vi "tack_point_builder.vi"(0 "Boat Location":T1 {"North" format="%#_10f"; "East" format="%#_8f"}, 1 "Loop counts":i32, 2 "Amount to extend tack waypoints (m)":dbl, 5 "Distance for tack to travel (m)":dbl, 7 "Tolerance (meters?)":dbl, 9 "Angle (Final leyline -> WP) (deg)":dbl, 11 "Angle (Other leyline -> WP) (deg)":dbl, 12 "Final leyline (deg)":dbl, 13 "Other leyline (deg)":dbl) -> (4 "Proposed WP array":refnum<class "Waypoint.lvclass">[](array[class]), 6 "Other leyline (deg)":dbl, 10 "Angle (Final leyline -> WP) (deg) OUT":dbl, 15 "Angle (Other leyline -> WP) (deg) OUT":dbl)   [LabVIEW 2013]
doc: "This VI takes the information to build a series of tack waypoints and makes a temporary array of the waypoints.\n\nTHIS VI ASSUMES THAT ANOTHER SHORT TACK WILL BE COMPLETED AFTER IT, IT ENDS ON 'OTHER LEYLINE', NOT FINAL LEYLINE'.s\n\nEric Schneider, September 2014"
uses:
  Data/TypeDefs/UTM Location.ctl
  Classes/Waypoint/Waypoint.lvclass
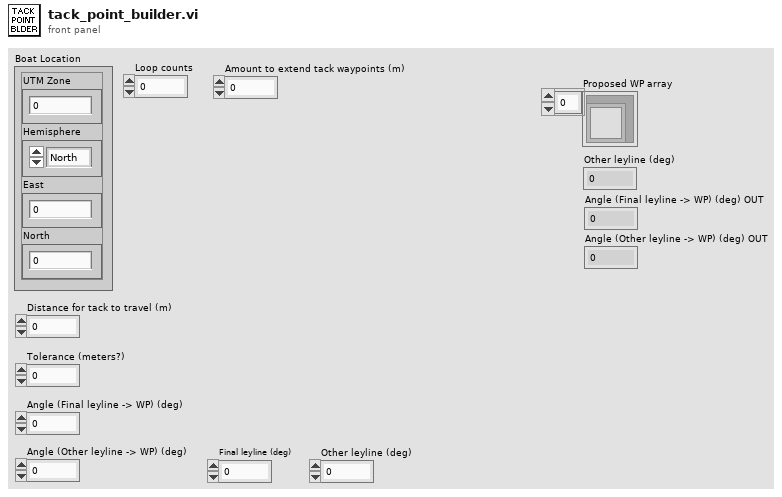
[diagram p1: front panel]
types:
  T1 = typedef "UTM Location.ctl" = cluster{"UTM Zone":dbl, "Hemisphere":enum16{"North", "South"}, "East":dbl, "North":dbl}
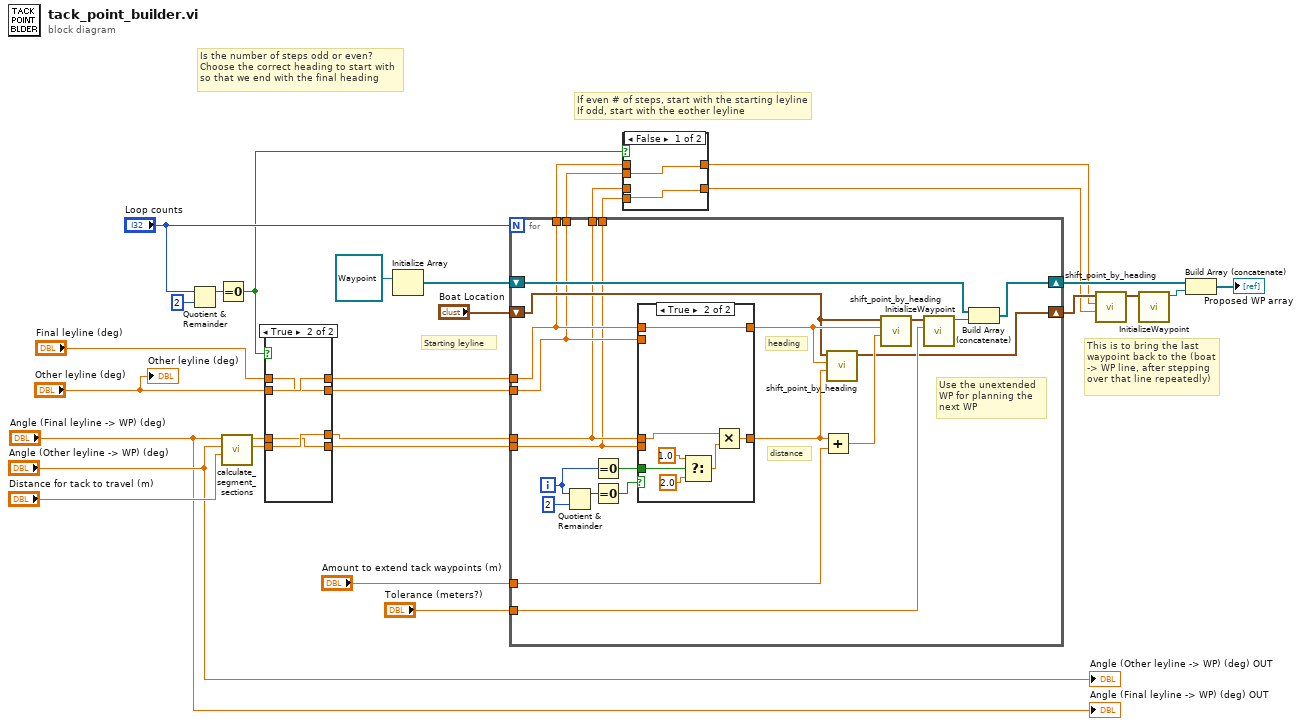
[diagram p0: block diagram]
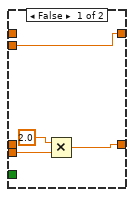
[diagram p4: hidden frame]
diagram:
  # "This is to bring the last waypoint back to the (boat -> WP line, after stepping over that line repeatedly)"
  # "If even # of steps, start with the starting leyline\nIf odd, start with the eother leyline"
  # "Starting leyline"
  # "Is the number of steps odd or even? Choose the correct heading to start with so that we end with the final heading"
  n1 = Quotient & Remainder(x="Loop counts", y=2) -> (x-y*floor(x/y)=w24:i32)  [unwired: 1 out]
  n2 = Equal To 0?(x=w24) -> (x = 0?=w12:bool)
  n3 = call "calculate_segment_sections.vi"("range (m)"="Distance for tack to travel (m)", "Angle WP to second leyline (deg)"="Angle (Other leyline -> WP) (deg)", "Angle WP to first leyline (deg)"="Angle (Final leyline -> WP) (deg)") -> ("Length of second leg (m)"=w15:dbl, "Length of first leg (m)"=w16:dbl)  [unwired: 5 in, 2 out]
  n4 = case shown="True" w12 {
    tunnel: "Final leyline (deg)" -> [w35 w38]
    tunnel: [w35 w39] -> w26
    tunnel: [w34 w38] -> w28
    tunnel: "Other leyline (deg)" -> [w34 w39]
    tunnel: w16 -> [w33 w36]
    tunnel: w15 -> [w32 w37]
    tunnel: [w33 w37] -> w14
    tunnel: [w32 w36] -> w13
    frame False {
    }
    frame True {
    }
  }
  n5 = Initialize Array(refnum<class "Waypoint.lvclass"> refnum ("element")) -> (w30:refnum<class "Waypoint.lvclass">[])  [unwired: 1 in]
  n6 = for {
    N: "Loop counts" -> [_]
    tunnel: w14 -> [w43]
    tunnel: w13 -> [w40]
    tunnel: w26 -> [w45]
    tunnel: w28 -> [w44]
    shift-right: [w52] -> w8
    shift-left: w30 -> [w54]
    tunnel: "Amount to extend tack waypoints (m)" -> [w50]
    tunnel: "Tolerance (meters?)" -> [w56]
    shift-right: [w48] -> w9
    shift-left: "Boat Location" -> [w49]
    tunnel: [w45] -> w6
    tunnel: [w44] -> w5
    tunnel: [w43] -> w4
    tunnel: [w40] -> w3
    i -> [w42]
    # "Use the unextended WP for planning the next WP"
    # "distance"
    # "heading"
    n7 = Quotient & Remainder(x=w42, y=2) -> (x-y*floor(x/y)=w58:i32)  [unwired: 1 out]
    n8 = Equal To 0?(x=w42) -> (x = 0?=w41:bool)
    n9 = Equal To 0?(x=w58) -> (x = 0?=w47:bool)
    n10 = case shown="True" w47 {
      tunnel: w45 -> [_ w70]
      tunnel: w44 -> [w63 _]
      tunnel: w43 -> [_ w68]
      tunnel: w40 -> [w61 _]
      tunnel: [w63 w70] -> w51
      tunnel: [w62 w69] -> w46
      tunnel: w41 -> [_ w67]
      frame False {
        n11 = Multiply(x=2.0, y=w61) -> (x*y=w62:dbl)
      }
      frame True {
        n12 = Select(t=1.0, s=w67, f=2.0 ("t")) -> (s? t:f=w66:dbl)
        n13 = Multiply(x=w68, y=w66) -> (x*y=w69:dbl)
      }
    }
    n14 = Add(x=w46, y=w50) -> (x+y=w53:dbl)
    n15 = call "shift_point_by_heading.vi"("Distance (m)"=w46, "Heading (deg)"=w51, "UTM Point"=w49) -> ("Shifted UTM Point"=w48:T1)  [unwired: 8 in]
    n16 = call "shift_point_by_heading.vi"("Distance (m)"=w53, "Heading (deg)"=w51, "UTM Point"=w49) -> ("Shifted UTM Point"=w57:T1)  [unwired: 8 in]
    n17 = call "InitializeWaypoint.vi"("Tolerance (meters?) (0)"=w56, "Coords"=w57) -> ("Waypoint Out"=w55:refnum<class "Waypoint.lvclass">)  [unwired: 9 in]
    n18 = Build Array (concatenate)(w54, w55) -> (w52:refnum<class "Waypoint.lvclass">[])
  }
  n19 = case shown="False" w12 {
    tunnel: w6 -> [_ w74]
    tunnel: w5 -> [w72 _]
    tunnel: [w72 w74] -> w2
    tunnel: w4 -> [_ w73]
    tunnel: w3 -> [w71 _]
    tunnel: [w71 w73] -> w1
    frame False {
    }
    frame True {
    }
  }
  n20 = call "shift_point_by_heading.vi"("Distance (m)"=w1, "Heading (deg)"=w2, "UTM Point"=w9) -> ("Shifted UTM Point"=w10:T1)  [unwired: 8 in]
  n21 = call "InitializeWaypoint.vi"("Coords"=w10) -> ("Waypoint Out"=w11:refnum<class "Waypoint.lvclass">)  [unwired: 10 in]
  n22 = Build Array (concatenate)(w8, w11) -> (→"Proposed WP array":refnum<class "Waypoint.lvclass">[])
  "Other leyline (deg)" <- "Other leyline (deg)"
  "Angle (Final leyline -> WP) (deg) OUT" <- "Angle (Final leyline -> WP) (deg)"
  "Angle (Other leyline -> WP) (deg) OUT" <- "Angle (Other leyline -> WP) (deg)"
